vi "get_error_kind.vi"(8 "error in (no error)":errorcluster, 11 "Request in":refnum<class "Request.lvclass">) -> (0 "error out":errorcluster, 2 "error_kind":T1, 3 "Request out":refnum<class "Request.lvclass">)   [LabVIEW 2020, in "reqwest.lvlib" / "Request.lvclass"]
uses:
  Request.lvclass
  reqwest_error_kind_enum.ctl
  Request.lvclass/Request.ctl
  lv_reqwest_64.so
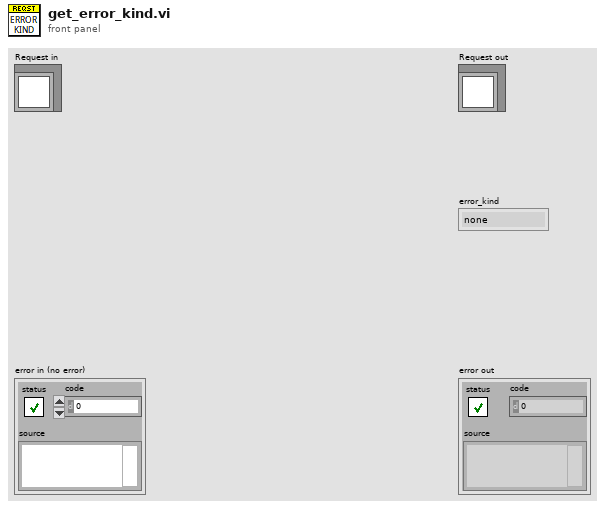
[diagram p1: front panel]
types:
  T1 = typedef "reqwest.lvlib/Request.lvclass/reqwest_error_kind_enum.ctl" = enum16{"none", "timeout", "connection", "redirect", "invalid_status", "body", "decode", "builder", "request", "file_system", "unknown"}
  T2 = typedef "reqwest.lvlib/Request.lvclass/request_id.ctl" = u64
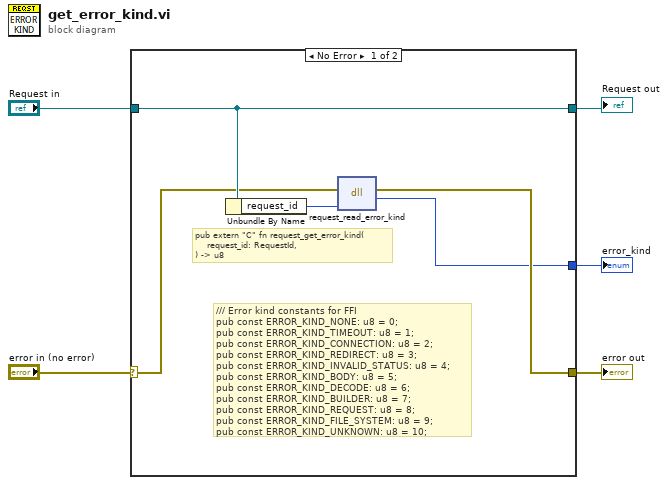
[diagram p0: block diagram]
diagram:
  n1 = case shown="No Error" "error in (no error)" {
    selector: "error in (no error)" -> [w8 w11]
    tunnel: "Request in" -> [w9 w12]
    tunnel: [w6 _] -> w3
    tunnel: [w10 w11] -> w1
    tunnel: [w9 w12] -> w2
    frame No Error {
      # "/// Error kind constants for FFI\npub const ERROR_KIND_NONE: u8 = 0;\npub const ERROR_KIND_TIMEOUT: u8 = 1;\npub const ERROR_KIND_CONNECTION: u8 = 2;\npub const ERROR_KIND_REDIRECT: u8 = 3;\npub const ERROR_KIND_INVALID_STATUS: u8 = 4;\npub const ERROR_KIND_BODY: u8 = 5;\npub const ERROR_KIND_DECODE: u8 = 6;\npub const ERROR_KIND_BUILDER: u8 = 7;\npub const ERROR_KIND_REQUEST: u8 = 8;\npub const ERROR_KIND_FILE_SYSTEM: u8 = 9;\npub const ERROR_KIND_UNKNOWN: u8 = 10;"
      # "pub extern \"C\" fn request_get_error_kind(\n    request_id: RequestId,\n) -> u8"
      n2 = Unbundle By Name(w9) -> ("request_id"=w7:T2)
      n3 = dll-call lib="home/jim-kring/Projects/reqwest-rs-labview/lv_src/lv_reqwest_*.*" fn="request_read_error_kind"(error in=w8, "request_id"=w7) -> (error out=w10:errorcluster, "error_kind"=w6:u8)  [unwired: 3 in, 1 out]
    }
    frame Error {
    }
  }
  "error out" <- w1
  "error_kind" <- w3
  "Request out" <- w2
